vi "SimpleMotorTest.vi"() -> ()   [LabVIEW 2011]
panel:
  out "MPL successful?":bool[](array[boolean])
  out "Position 2":dbl[](array[numeric]) format="%.6f"
  in  "String":string
  out "Conn. Axes out":string[](array[string])
  out "+/- movement\nrange":dbl[](array[numeric]) format="%.6f"
  in  "System no.":i32=1 min=1 step=1
  in  "Stage names input":string[](array[string])=["M-126.PD", "C-150.PD"]
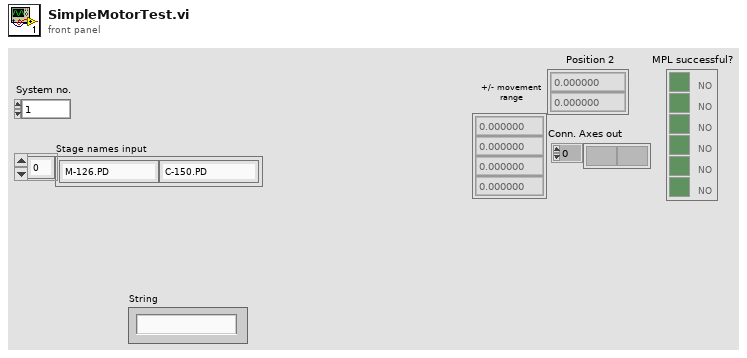
[diagram p1: front panel]
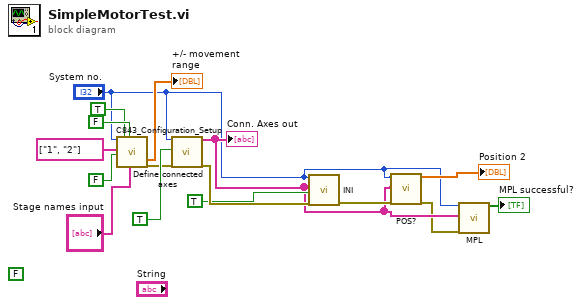
[diagram p0: block diagram]
diagram:
  (unwired) FALSE ("All axes?")
  n1 = call "C843_Configuration_Setup.vi"("System no."="System no.", "Axes to move"=string[] ["1", "2"] ("Axes to query"), "All axes?"=FALSE, "C-843 version"=TRUE, "Use dialog to define\nconnected stages?"=FALSE ("Use dialog to define\nconnected stages?"), "Stage names input"="Stage names input") -> ("+/- movement\nrange"=→"+/- movement\nrange":dbl[], "error out"=w11:errorcluster)  [unwired: 9 in, 3 out]
  n2 = call "Define connected axes.vi"("System no."="System no.", "Read from\ncontroller?"=TRUE ("Read from\ncontroller?"), "error in"=w11) -> ("Conn. Axes out"=w4:string[], "error out"=w10:errorcluster)  [unwired: 15 in]
  "Conn. Axes out" <- w4
  n3 = call "INI.vi"("System no."="System no.", "INI axes"=w4, "All axes?"=TRUE, "error in"=w10) -> ("error out"=w6:errorcluster)  [unwired: 15 in]
  n4 = call "POS?.vi"("System no."="System no.", "Axes to query"=w4, "error in"=w6) -> ("Position"=→"Position 2":dbl[], "error out"=w2:errorcluster)  [unwired: 15 in]
  n5 = call "MPL.vi"("System no."="System no.", "Affected axes"=w4, "error in"=w2) -> ("MPL successful?"=→"MPL successful?":bool[])  [unwired: 15 in, 1 out]
